vi "Array.vi"() -> ()   [LabVIEW 2021]
panel:
  in  "Rows":dbl=6.0
  out "Third Row Fifth Column":dbl
  out "Second Column":dbl[](array[numeric])
  out "Third row":dbl[](array[numeric])
  in  "Columns":dbl
  out "Array":dbl[][](array[numeric])
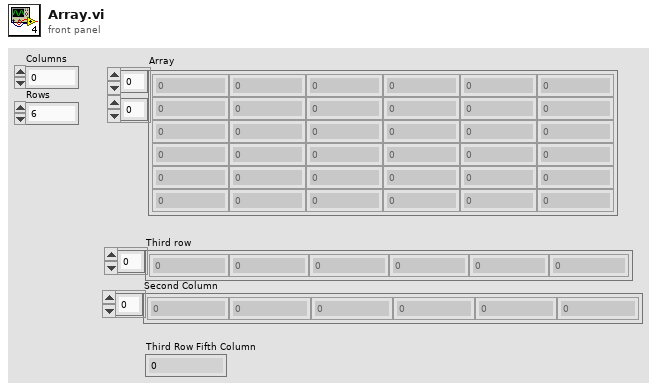
[diagram p1: front panel]
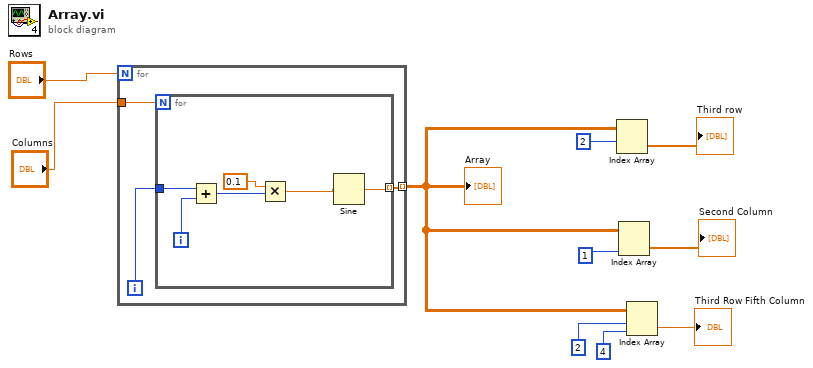
[diagram p0: block diagram]
diagram:
  n1 = for {
    N: "Rows" -> [_]
    tunnel: [w12] -> w1 mode=indexing
    tunnel: "Columns" -> [w11]
    i -> [w13]
    n2 = for {
      N: w11 -> [_]
      tunnel: w13 -> [w18]
      tunnel: [w14] -> w12 mode=indexing
      i -> [w19]
      n3 = Add(x=w18, y=w19) -> (x+y=w17:i32)
      n4 = Multiply(x=0.1, y=w17) -> (x*y=w15:dbl)
      n5 = Sine(x=w15) -> (sin(x)=w14:dbl)
    }
  }
  "Array" <- w1
  n6 = Index Array(array=w1, index (row)=2) -> (element=→"Third row":dbl[])  [unwired: 1 in]
  n7 = Index Array(array=w1, index (col)=1) -> (element=→"Second Column":dbl[])  [unwired: 1 in]
  n8 = Index Array(array=w1, index (row)=2, index (col)=4) -> (element=→"Third Row Fifth Column":dbl)
